vi "PAM Acquire Spectra TCP.vi"(10 "Spectrum ID":refnum<k5>) -> (2 "Timestamp Out":timestamp, 3 "PSD Out":dbl[](array[numeric]))   [LabVIEW 2020]
uses:
  PAM uPa per Bit.vi
  PAM Library.lvlib
panel:
  out "concatenated string":string
  in  "Unix Time":u32
  out "Time":timestamp
  out "data out":string
  out "Error Out":errorcluster
  out "Error Out":errorcluster
  out "Error Out":errorcluster
  out "Error Out":errorcluster
  out "Error Out":errorcluster
  out "Error Out":errorcluster
  out "Error Out":errorcluster
  out "Error Out":errorcluster
  out "Notification":string
  out "Data Header":string
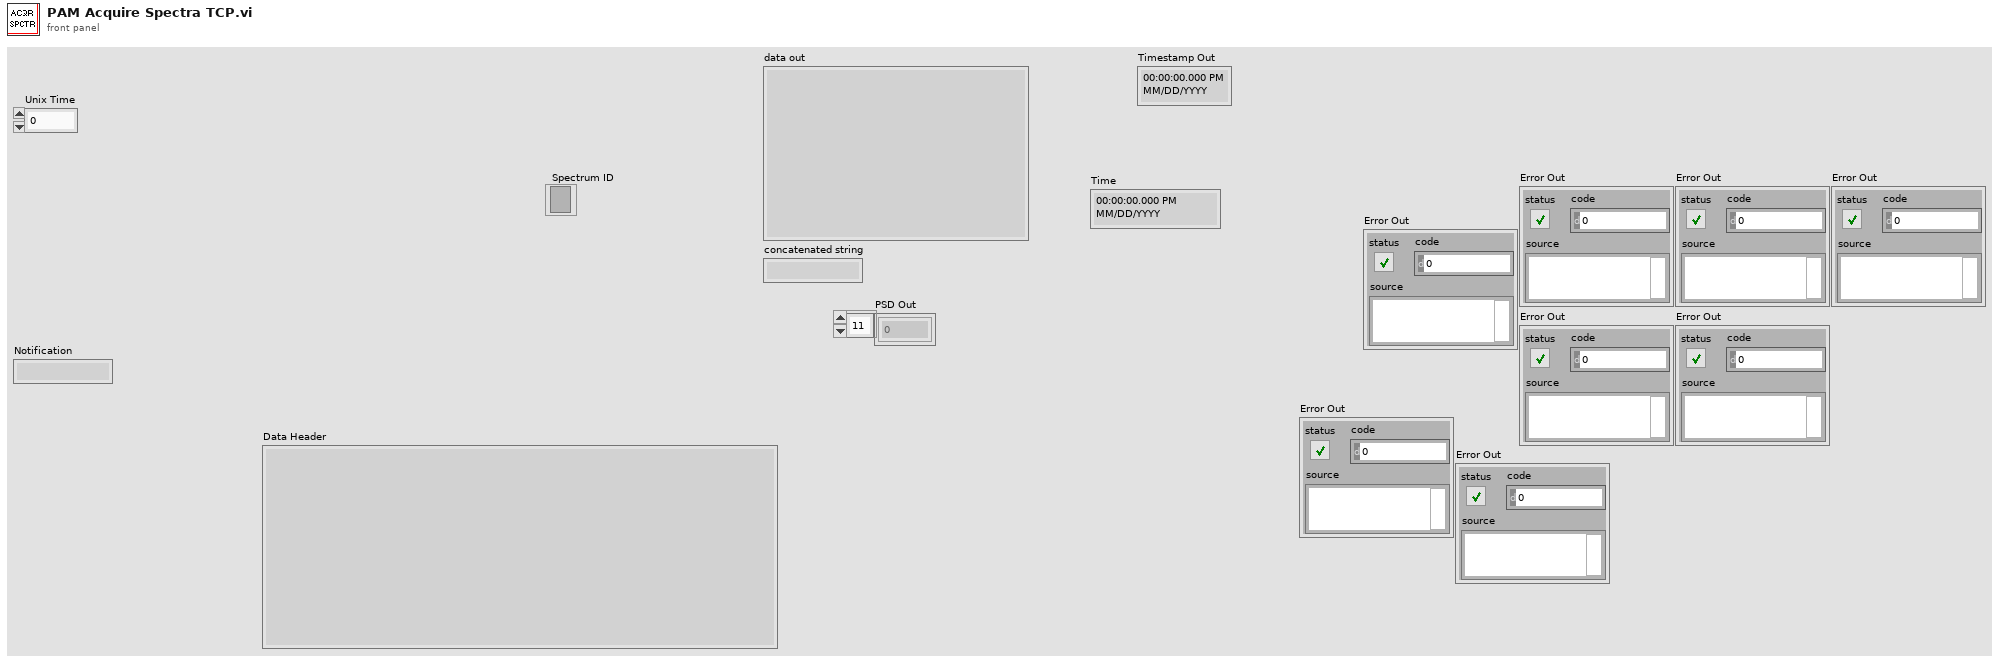
[diagram p1: front panel]
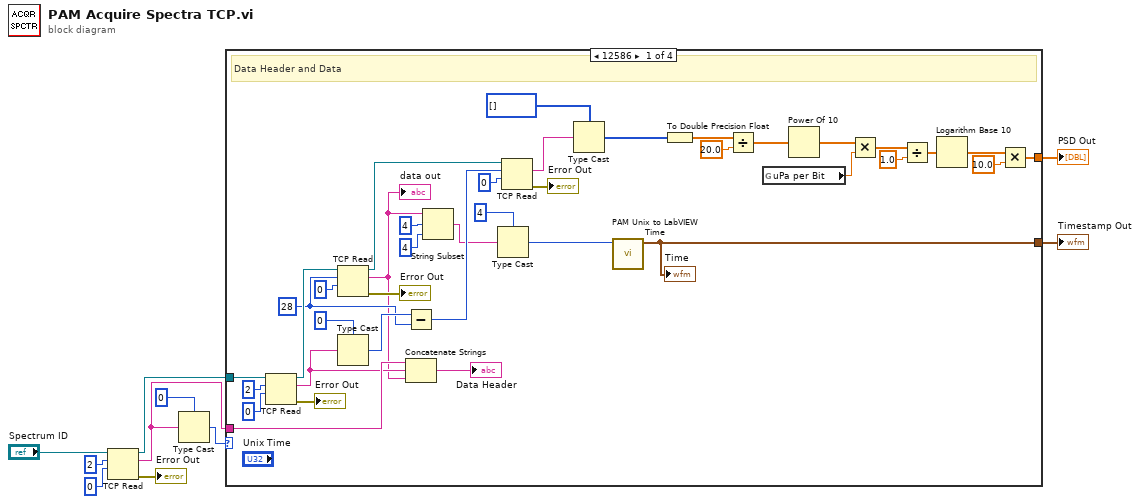
[diagram p0: block diagram]
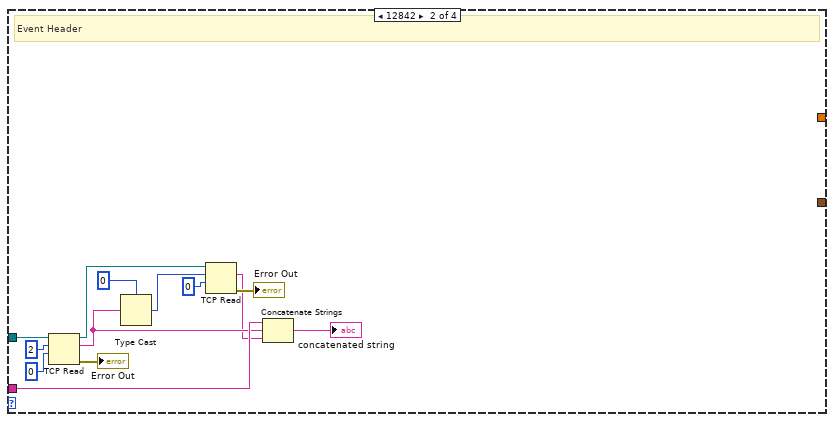
[diagram p2: hidden frame]
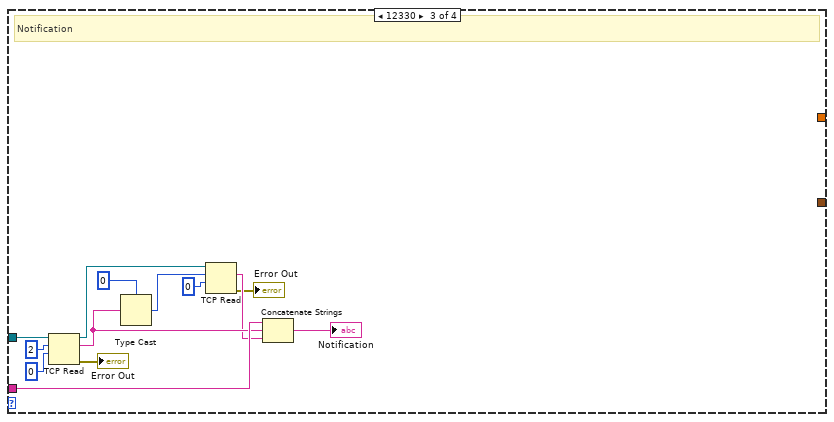
[diagram p3: hidden frame]
diagram:
  n1 = TCP Read(connection ID="Spectrum ID", bytes to read=2, 9:0 ("timeout ms (25000)")) -> (connection ID out=w6:refnum<k5>, data out=w7:string, error out=→"Error Out":errorcluster)  [unwired: 2 in]
  n2 = Type Cast(type=u16 0, x=w7) -> (*(type *) &x=w8:u16)
  n3 = case shown="12586" w8 {
    tunnel: w7 -> [w34 w60 w73 _]
    tunnel: w6 -> [w31 w59 w70 _]
    tunnel: [w19 _ _ _] -> w2
    tunnel: [w11 _ _ _] -> w1
    frame 12586 {
      w23 = u16 28
      # "Data Header and Data"
      n4 = TCP Read(connection ID=w31, bytes to read=u32 2 ("byte count"), 9:0 ("timeout ms (25000)")) -> (connection ID out=w29:refnum<k5>, data out=w25:string, error out=→"Error Out":errorcluster)  [unwired: 2 in]
      n5 = TCP Read(connection ID=w29, bytes to read=w23, 9:0 ("timeout ms (25000)")) -> (connection ID out=w28:refnum<k5>, data out=w18:string, error out=→"Error Out":errorcluster)  [unwired: 2 in]
      "data out" <- w18
      n6 = Type Cast(type=u16 0, x=w25) -> (*(type *) &x=w47:u16)
      n7 = Subtract(x=w47, y=w23) -> (x-y=w22:u16)
      n8 = Concatenate Strings(w34, w25, w18) -> (→"Data Header":string)
      n9 = String Subset(string=w18, offset (0)=4, length (rest)=4 ("length (rest)")) -> (substring=w15:string)
      n10 = Type Cast(type=u32 4 ("length (rest)"), x=w15) -> (*(type *) &x=w13:u32)
      n11 = TCP Read(connection ID=w28, bytes to read=w22, 9:0 ("timeout ms (25000)")) -> (data out=w24:string, error out=→"Error Out":errorcluster)  [unwired: 2 in, 1 out]
      n12 = Type Cast(type=u8[] [], x=w24) -> (*(type *) &x=w43:u8[])
      n13 = call "PAM Unix to LabVIEW Time.vi"("Unix"=w13) -> ("Labview Timestamp"=w11:timestamp)  [unwired: 10 in]
      "Time" <- w11
      n14 = To Double Precision Float(number=w43) -> (double precision float=w38:dbl[])
      n15 = Divide(x=w38, y=20.0) -> (x/y=w39:dbl[])
      n16 = global read "PAM uPa per Bit.vi" "uPa per Bit"() -> (w36:dbl)
      n17 = Power Of 10(x=w39) -> (10^x=w37:dbl[])
      n18 = Multiply(x=w37, y=w36) -> (x*y=w35:dbl[])
      n19 = Divide(x=w35, y=1.0) -> (x/y=w41:dbl[])
      n20 = Logarithm Base 10(1:w41) -> (0:w45:dbl[])
      n21 = Multiply(x=w45, y=10.0) -> (x*y=w19:dbl[])
    }
    frame 12842 {
      # "Event Header"
      n22 = TCP Read(connection ID=w59, bytes to read=u32 2 ("byte count"), 9:0 ("timeout ms (25000)")) -> (connection ID out=w54:refnum<k5>, data out=w55:string, error out=→"Error Out":errorcluster)  [unwired: 2 in]
      n23 = Type Cast(type=u16 0, x=w55) -> (*(type *) &x=w52:u16)
      n24 = TCP Read(connection ID=w54, bytes to read=w52, 9:0 ("timeout ms (25000)")) -> (data out=w50:string, error out=→"Error Out":errorcluster)  [unwired: 2 in, 1 out]
      n25 = Concatenate Strings(w60, w55, w50) -> (→"concatenated string":string)
    }
    frame 12330 {
      # "Notification"
      n26 = TCP Read(connection ID=w70, bytes to read=2 ("byte count"), 9:0 ("timeout ms (25000)")) -> (connection ID out=w68:refnum<k5>, data out=w69:string, error out=→"Error Out":errorcluster)  [unwired: 2 in]
      n27 = Type Cast(type=u16 0, x=w69) -> (*(type *) &x=w67:u16)
      n28 = TCP Read(connection ID=w68, bytes to read=w67, 9:0 ("timeout ms (25000)")) -> (data out=w64:string, error out=→"Error Out":errorcluster)  [unwired: 2 in, 1 out]
      n29 = Concatenate Strings(w73, w69, w64) -> (→"Notification":string)
    }
    frame 0, Default {
    }
  }
  "PSD Out" <- w2
  "Timestamp Out" <- w1
